vi "main.vi"(8 "error in (no error)":errorcluster, 11 "functional":refnum<user-event>) -> (0 "error out":errorcluster)   [LabVIEW 2015, in "functional.lvlib"]
uses:
  functional.lvlib
  _controls/event_functional.ctl
  _controls/event_functional_command.ctl
  private/_controls/event_common.ctl
  private/_controls/event_common_command.ctl
  private/_controls/event_interface.ctl
  private/_controls/event_interface_command.ctl
  _controls/hmi_references.ctl
  examples/example_01/functional/public/interface/interface.lvclass
  _controls/menu_selection.ctl
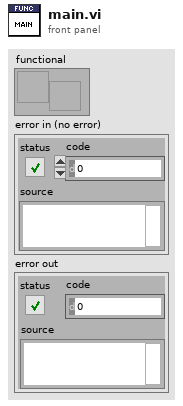
[diagram p1: front panel]
types:
  T1 = typedef "functional.lvlib/event_interface.ctl" = cluster{"command":T2, "data":variant}
  T2 = typedef "functional.lvlib/event_interface_command.ctl" = enum16{"<event_interface_cmd>", "<null>"}
  T3 = typedef "functional.lvlib/event_common.ctl" = cluster{"command":T4, "data":variant}
  T4 = typedef "functional.lvlib/event_common_command.ctl" = enum16{"<event_common_cmd>", "update_hmi_references", "die", "<null>"}
  T5 = cluster{"local":refnum<event-registration>, "external":refnum<event-registration>}
  T6 = typedef "functional.lvlib/hmi_references.ctl" = cluster{"vi_reference":refnum<vi>, "random_number":refnum<vi>, "do_it":refnum<vi>}
  T7 = cluster{"queue out":refnum<queue>, "example_01.lvlib:functional.lvlib:interface.lvclass":refnum<class "interface.lvclass">}
  T8 = typedef "functional.lvlib/event_functional.ctl" = cluster{"command":T9, "data":variant}
  T9 = typedef "functional.lvlib/event_functional_command.ctl" = enum16{"<command_functional>", "--high-level", "stop", "update_hmi_references", "load_interface", "--functional", "do_it", "<null>"}
  T10 = typedef "functional.lvlib/menu_selection.ctl" = enum16{"<menu>", "file_exit", "help_about", "<null>"}
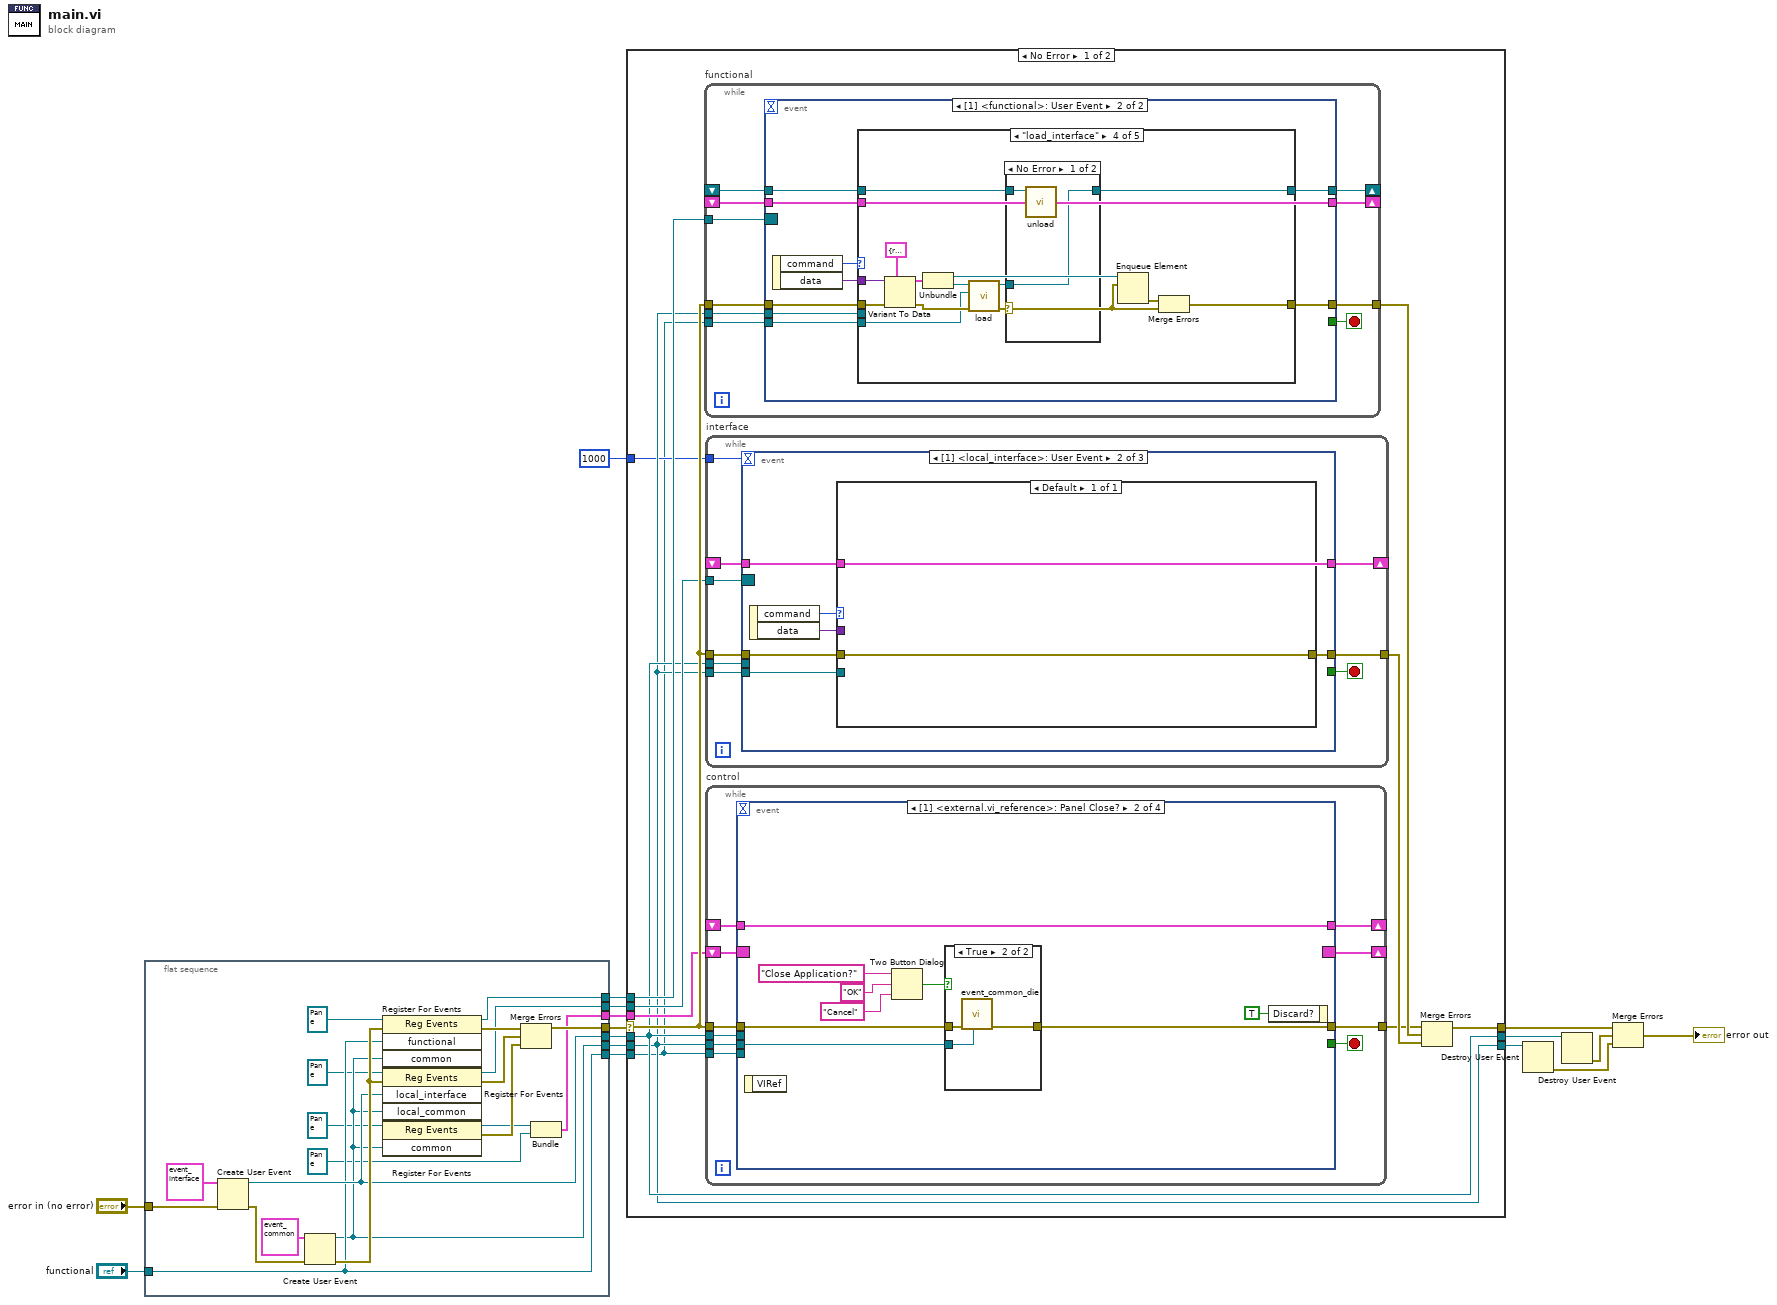
[diagram p0: block diagram]
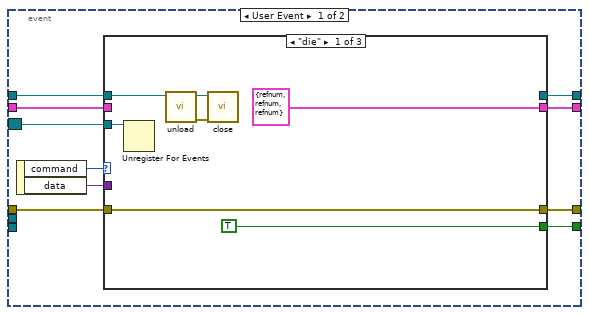
[diagram p2: hidden frame]
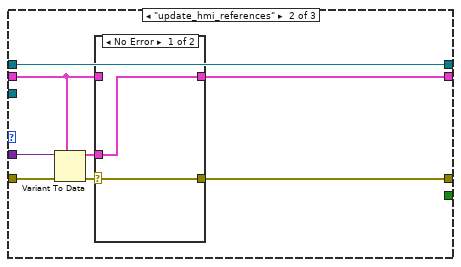
[diagram p3: hidden frame]
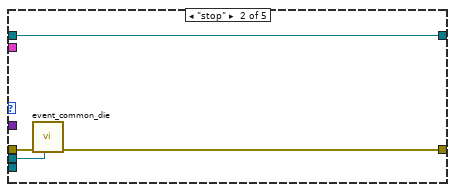
[diagram p7: hidden frame]
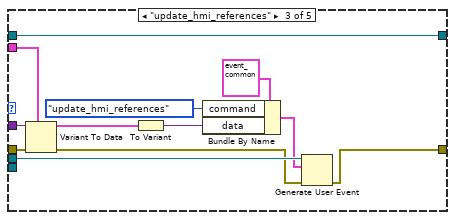
[diagram p8: hidden frame]
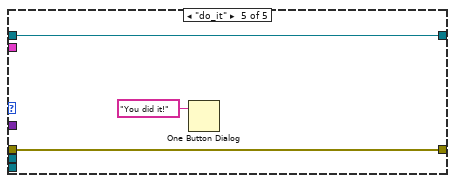
[diagram p10: hidden frame]
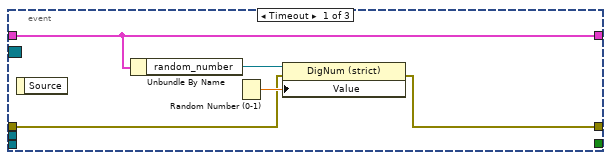
[diagram p11: hidden frame]
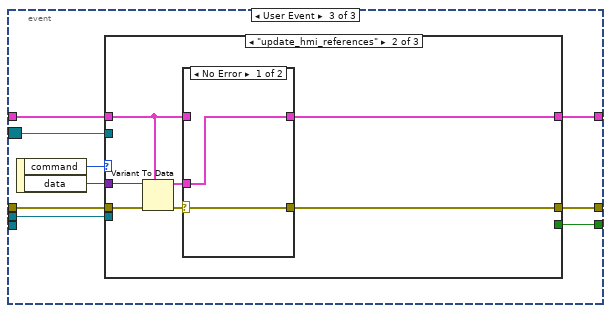
[diagram p12: hidden frame]
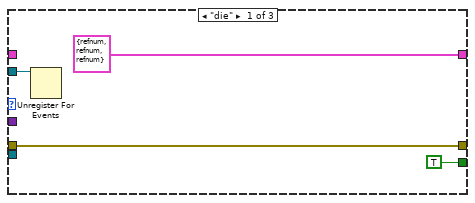
[diagram p13: hidden frame]
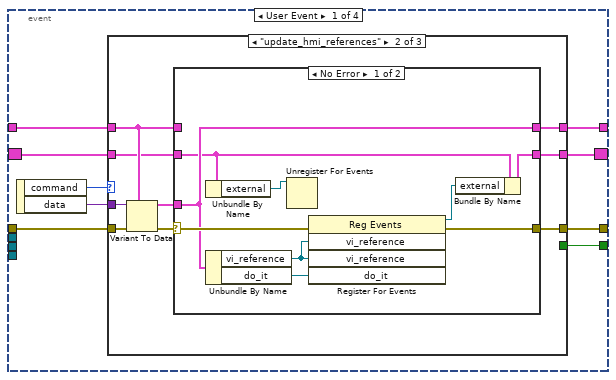
[diagram p16: hidden frame]
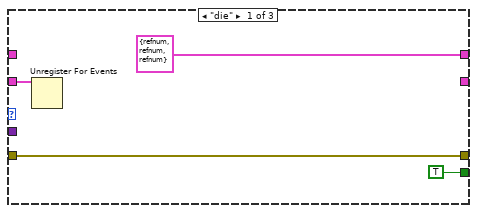
[diagram p17: hidden frame]
diagram:
  n1 = flat-sequence {
    tunnel: [w31] -> w16
    tunnel: [w21] -> w15
    tunnel: "error in (no error)" -> [w26]
    tunnel: [w30] -> w13
    tunnel: [w23] -> w11
    tunnel: [w27] -> w12
    tunnel: "functional" -> [w25]
    tunnel: [w25] -> w3
    tunnel: [w24] -> w2
    frame #0 {
      n2 = Create User Event(user event datatype=T1 {"command"=enum."<event_interface_cmd>", "data"=variant} ("interface"), error in=w26) -> (user event=w27:refnum<user-event>, error out=w32:errorcluster)
      n3 = Create User Event(user event datatype=T3 {"command"=enum."<event_common_cmd>", "data"=variant} ("common"), error in=w32) -> (user event=w23:refnum<user-event>, error out=w33:errorcluster)
      n4 = register-events(reference=refnum<event-registration> refnum ("local"), error in=w33, w25, w23) -> (reference out=w24:refnum<event-registration>, error out=w34:errorcluster)
      n5 = register-events(reference=refnum<event-registration> refnum ("local"), error in=w33, w27, w23) -> (reference out=w30:refnum<event-registration>, error out=w35:errorcluster)
      n6 = register-events(reference=refnum<event-registration> refnum ("local"), w23) -> (reference out=w22:refnum<event-registration>, error out=w36:errorcluster)  [unwired: 1 in]
      n7 = Merge Errors(w34, w35, w36) -> (w31:errorcluster)
      n8 = Bundle("local"=w22, "external"=refnum<event-registration> refnum) -> (w21:T5)  [unwired: 1 in]
    }
  }
  n9 = case shown="No Error" w16 {
    selector: w16 -> [w47 w279]
    tunnel: w15 -> [w45 w275]
    tunnel: [w43 w279] -> w8
    tunnel: w13 -> [w44 w276]
    tunnel: w12 -> [w42 w278]
    tunnel: w11 -> [w41 w277]
    tunnel: [w42 w278] -> w9
    tunnel: [w41 w277] -> w10
    tunnel: w3 -> [w37 _]
    tunnel: w2 -> [w48 w274]
    tunnel: 1000 -> [w38 _]
    frame No Error {
      n10 = while "functional" {
        tunnel: [w58] -> w40
        tunnel: w47 -> [w57]
        tunnel: w48 -> [w56]
        tunnel: w41 -> [w53]
        shift-right: [w52] -> _
        shift-left: _ -> [w55]
        tunnel: w37 -> [w51]
        shift-right: [w49] -> _
        shift-left: _ -> [w50]
        stop <- w54 stop-if-true
        n11 = event shown="[1] <functional>: User Event" {
          selector: w56 -> [w68 _]
          dyn-events: _ -> [_ _]
          timeout: _ -> [_ _]
          tunnel: [w65 w96] -> w58
          tunnel: w57 -> [w66 w97]
          tunnel: w55 -> [w62 w94]
          tunnel: [w64 _] -> w54
          tunnel: w53 -> [_ w95]
          tunnel: [w61 w94] -> w52
          tunnel: w51 -> [_ w93]
          tunnel: w50 -> [w60 w92]
          tunnel: [w59 w91] -> w49
          event User Event {
            n12 = event-data() -> ("command"=w67:T4, "data"=w63:variant)  [unwired: 1 in]
            n13 = case shown="\"die\"" w67 {
              tunnel: w66 -> [w74 w82 w90]
              tunnel: [w74 w80 w90] -> w65
              tunnel: [TRUE _ _] -> w64
              tunnel: w68 -> [w73 _ _]
              tunnel: w63 -> [_ w83 _]
              tunnel: w62 -> [_ w79 w89]
              tunnel: [T6 {"vi_reference"=refnum, "random_number"=refnum, "do_it"=refnum} ("hmi_references") w77 w89] -> w61
              tunnel: w60 -> [w71 w76 w88]
              tunnel: [_ w76 w88] -> w59
              frame "die" {
                n14 = Unregister For Events(event registration refnum=w73) -> ()  [unwired: 1 in, 1 out]
                n15 = call-dynamic "unload.vi"("interface in"=w71) -> ("error out"=w69:errorcluster, "interface out"=w70:refnum<class "interface.lvclass">)  [unwired: 9 in]
                n16 = call-dynamic "close.vi"("error in (no error)"=w69, "interface in"=w70) -> ()  [unwired: 8 in, 2 out]
              }
              frame "update_hmi_references" {
                n17 = Variant To Data(error in=w82, type=w79, Variant=w83) -> (data=w78:T6, error out=w81:errorcluster)
                n18 = case shown="No Error" w81 {
                  selector: w81 -> [w85 w87]
                  tunnel: [w85 w87] -> w80
                  tunnel: w79 -> [_ w86]
                  tunnel: w78 -> [w84 _]
                  tunnel: [w84 w86] -> w77
                  frame No Error {
                  }
                  frame Error {
                  }
                }
              }
              frame Default {
              }
            }
          }
          event User Event {
            n19 = event-data() -> ("command"=w98:T9, "data"=w99:variant)  [unwired: 1 in]
            n20 = case shown="\"load_interface\"" w98 {
              tunnel: w99 -> [_ _ w112 w130 _]
              tunnel: w97 -> [w101 w103 w117 w131 w137]
              tunnel: [w101 w102 w114 w122 w137] -> w96
              tunnel: w95 -> [_ w104 w116 _ _]
              tunnel: w94 -> [_ _ w113 _ _]
              tunnel: w93 -> [_ _ _ w127 _]
              tunnel: w92 -> [w100 w105 w106 w126 w135]
              tunnel: [w100 w105 w106 w118 w135] -> w91
              frame Default {
              }
              frame "stop" {
                n21 = call "event_common_die.vi"("local_common"=w104, "error in (no error)"=w103) -> ("error out"=w102:errorcluster)  [unwired: 9 in]
              }
              frame "update_hmi_references" {
                n22 = Variant To Data(error in=w117, type=w113, Variant=w112) -> (data=w109:T6, error out=w115:errorcluster)
                n23 = To Variant(anything=w109) -> (Variant=w107:variant)
                n24 = Bundle By Name(cluster=T3 {"command"=enum."<event_common_cmd>", "data"=variant} ("event data"), "command"=event_common_command."update_hmi_references", "data"=w107) -> (w110:T3)
                n25 = Generate User Event(user event=w116, event data cluster=w110, error in=w115) -> (error out=w114:errorcluster)  [unwired: 1 in, 1 out]
              }
              frame "load_interface" {
                n26 = Variant To Data(error in=w131, type=T7 {"queue out"=refnum, "example_01.lvlib:functional.lvlib:interface.lvclass"=refnum}, Variant=w130) -> (data=w129:T7, error out=w128:errorcluster)
                n27 = Unbundle(w129) -> ("queue out"=w123:refnum<queue>, "example_01.lvlib:functional.lvlib:interface.lvclass"=w124:refnum<class "interface.lvclass">)
                n28 = call-dynamic "load.vi"("error in (no error)"=w128, "functional"=w127, "interface in"=w124) -> ("error out"=w120:errorcluster, "interface out"=w119:refnum<class "interface.lvclass">)  [unwired: 7 in]
                n29 = case shown="No Error" w120 {
                  tunnel: w126 -> [w133 w134]
                  tunnel: w119 -> [w132 _]
                  tunnel: [w132 w134] -> w118
                  frame No Error {
                    n30 = call-dynamic "unload.vi"("interface in"=w133) -> ()  [unwired: 9 in, 2 out]
                  }
                  frame Error {
                  }
                }
                n31 = Enqueue Element(queue=w123, element=w120) -> (error out=w121:errorcluster)  [unwired: 2 in, 2 out]
                n32 = Merge Errors(w121, w120) -> (w122:errorcluster)
              }
              frame "do_it" {
                n33 = One Button Dialog(message="You did it!") -> ()  [unwired: 1 in, 1 out]
              }
            }
          }
        }
      }
      n34 = while "interface" {
        tunnel: w47 -> [w146]
        tunnel: [w144] -> w46
        tunnel: w44 -> [w143]
        tunnel: w42 -> [w138]
        tunnel: w41 -> [w142]
        shift-right: [w140] -> _
        shift-left: _ -> [w141]
        tunnel: w38 -> [w139]
        stop <- w145 stop-if-true
        n35 = event shown="[1] <local_interface>: User Event" {
          selector: w143 -> [_ _ w163]
          dyn-events: _ -> [_ _ _]
          timeout: w139 -> [_ _ _]
          tunnel: w146 -> [w148 w155 w166]
          tunnel: [w147 w154 w165] -> w144
          tunnel: [_ _ w164] -> w145
          tunnel: w142 -> [_ w153 _]
          tunnel: w141 -> [w149 w152 w161]
          tunnel: [w149 w152 w160] -> w140
          tunnel: w138 -> [_ _ w159]
          event Timeout {
            n36 = event-data() -> ()  [unwired: 1 in, 1 out]
            n37 = Unbundle By Name(w149) -> ("random_number"=w151:refnum<vi>)
            n38 = Random Number (0-1)() -> (number: 0 to 1=w150:dbl)
            n39 = property class="DigNum (strict)"(reference=w151, error in=w148, "Value"=w150) -> (error out=w147:errorcluster)  [unwired: 1 out]
          }
          event User Event {
            n40 = event-data() -> ("command"=w157:T2, "data"=w156:variant)  [unwired: 1 in]
            n41 = case shown="Default" w157 {
              tunnel: w155 -> [w158]
              tunnel: [w158] -> w154
              tunnel: w156 -> [_]
              tunnel: w153 -> [_]
              tunnel: w152 -> [_]
              frame Default {
              }
            }
          }
          event User Event {
            n42 = event-data() -> ("command"=w167:T4, "data"=w162:variant)  [unwired: 1 in]
            n43 = case shown="\"update_hmi_references\"" w167 {
              tunnel: w166 -> [w170 w175 w184]
              tunnel: [w170 w172 w184] -> w165
              tunnel: [TRUE _ _] -> w164
              tunnel: w163 -> [w169 _ _]
              tunnel: w162 -> [_ w174 _]
              tunnel: w161 -> [_ w176 w183]
              tunnel: [T6 {"vi_reference"=refnum, "random_number"=refnum, "do_it"=refnum} ("hmi_references") w173 w183] -> w160
              tunnel: w159 -> [_ _ _]
              frame "die" {
                n44 = Unregister For Events(event registration refnum=w169) -> ()  [unwired: 1 in, 1 out]
              }
              frame "update_hmi_references" {
                n45 = Variant To Data(error in=w175, type=w176, Variant=w174) -> (data=w177:T6, error out=w178:errorcluster)
                n46 = case shown="No Error" w178 {
                  selector: w178 -> [w179 w182]
                  tunnel: [w179 w182] -> w172
                  tunnel: w176 -> [_ w181]
                  tunnel: w177 -> [w180 _]
                  tunnel: [w180 w181] -> w173
                  frame No Error {
                  }
                  frame Error {
                  }
                }
              }
              frame Default {
              }
            }
          }
        }
      }
      n47 = while "control" {
        tunnel: w47 -> [w194]
        tunnel: [w192] -> w39
        tunnel: w42 -> [w189]
        tunnel: w41 -> [w188]
        shift-right: [w187] -> _
        shift-left: _ -> [w190]
        shift-right: [w186] -> _
        shift-left: w45 -> [w191]
        tunnel: w37 -> [w185]
        stop <- w193 stop-if-true
        n48 = event shown="[1] <external.vi_reference>: Panel Close?" {
          selector: w191 -> [w198 _ _ _]
          dyn-events: [w195 _ _ _] -> w186
          timeout: _ -> [_ _ _ _]
          tunnel: w194 -> [w202 w234 w247 w254]
          tunnel: [w201 w239 w246 w252] -> w192
          tunnel: [w200 _ _ _] -> w193
          tunnel: w190 -> [w197 w233 w249 w251]
          tunnel: w189 -> [_ _ _ _]
          tunnel: w188 -> [_ w232 _ w250]
          tunnel: [w196 w233 w249 w251] -> w187
          tunnel: w185 -> [_ _ w248 _]
          event User Event {
            n49 = event-data() -> ("command"=w203:T4, "data"=w199:variant)  [unwired: 1 in]
            n50 = case shown="\"update_hmi_references\"" w203 {
              tunnel: w202 -> [w205 w212 w231]
              tunnel: [w205 w210 w231] -> w201
              tunnel: [TRUE _ _] -> w200
              tunnel: w199 -> [_ w214 _]
              tunnel: w198 -> [w206 w209 w230]
              tunnel: w197 -> [_ w213 w229]
              tunnel: [T6 {"vi_reference"=refnum, "random_number"=refnum, "do_it"=refnum} ("hmi_references") w211 w229] -> w196
              tunnel: [_ w208 w230] -> w195
              frame "die" {
                n51 = Unregister For Events(event registration refnum=w206) -> ()  [unwired: 1 in, 1 out]
              }
              frame "update_hmi_references" {
                n52 = Variant To Data(error in=w212, type=w213, Variant=w214) -> (data=w216:T6, error out=w215:errorcluster)
                n53 = case shown="No Error" w215 {
                  selector: w215 -> [w223 w228]
                  tunnel: [w222 w228] -> w210
                  tunnel: w213 -> [_ w227]
                  tunnel: w216 -> [w220 _]
                  tunnel: [w220 w227] -> w211
                  tunnel: w209 -> [w218 w226]
                  tunnel: [w225 w226] -> w208
                  frame No Error {
                    n54 = Unbundle By Name(w218) -> ("external"=w217:refnum<event-registration>)
                    n55 = Unbundle By Name(w220) -> ("vi_reference"=w219:refnum<vi>, "do_it"=w224:refnum<vi>)
                    n56 = Unregister For Events(event registration refnum=w217) -> ()  [unwired: 1 in, 1 out]
                    n57 = register-events(error in=w223, w219, w219, w224) -> (reference out=w221:refnum<event-registration>, error out=w222:errorcluster)  [unwired: 1 in]
                    n58 = Bundle By Name(cluster=w218, "external"=w221) -> (w225:T5)
                  }
                  frame Error {
                  }
                }
              }
              frame Default {
              }
            }
          }
          event Panel Close? {
            n59 = event-data() -> ()  [unwired: 1 in, 1 out]
            n60 = Two Button Dialog(message="Close Application?" ("dialog_text"), 1:"Cancel" ("boolean_text_1"), 2:"OK" ("boolean_text_1")) -> (T button?=w235:bool)
            n61 = case shown="True" w235 {
              tunnel: w234 -> [w241 w243]
              tunnel: [w241 w242] -> w239
              tunnel: w232 -> [_ w244]
              frame False {
              }
              frame True {
                n62 = call "event_common_die.vi"("local_common"=w244, "error in (no error)"=w243) -> ("error out"=w242:errorcluster)  [unwired: 9 in]
              }
            }
            n63 = event-data("Discard?"=TRUE) -> ()  [unwired: 1 in, 1 out]
          }
          event Value Change {
            n64 = event-data() -> ()  [unwired: 1 in, 1 out]
            n65 = Generate User Event(user event=w248, event data cluster=T8 {"command"=enum."do_it", "data"=variant} ("event data"), error in=w247) -> (error out=w246:errorcluster)  [unwired: 1 in, 1 out]
          }
          event Menu Selection (User) {
            n66 = event-data() -> ("MenuRef"=w255:refnum<k9>, "ItemTag"=w253:string)  [unwired: 1 in]
            n67 = Scan From String(input string=w253, default 1=menu_selection."<menu>" ("menu_selection")) -> (output 1=w256:T10)  [unwired: 3 in, 3 out]
            n68 = case shown="\"file_exit\"" w256 {
              tunnel: w255 -> [_ _]
              tunnel: w254 -> [w258 w263]
              tunnel: w253 -> [w262 _]
              tunnel: [w258 w269] -> w252
              tunnel: w250 -> [_ w268]
              frame Default {
                n69 = Format Into String(format string="Invalid Menu Option Selected: %s.", w262) -> (resulting string=w260:string)  [unwired: 2 in, 1 out]
                n70 = One Button Dialog(message=w260, button name ("OK")="OK" ("boolean_text_1")) -> ()  [unwired: 1 out]
              }
              frame "file_exit" {
                n71 = Two Button Dialog(message="Close Application?" ("dialog_text"), 1:"Cancel" ("boolean_text_1"), 2:"OK" ("boolean_text_1")) -> (T button?=w264:bool)
                n72 = case shown="False" w264 {
                  tunnel: w263 -> [w270 w273]
                  tunnel: [w270 w272] -> w269
                  tunnel: w268 -> [_ w271]
                  frame False {
                  }
                  frame True {
                    n73 = call "event_common_die.vi"("local_common"=w271, "error in (no error)"=w273) -> ("error out"=w272:errorcluster)  [unwired: 9 in]
                  }
                }
              }
            }
          }
        }
      }
      n74 = Merge Errors(w39, w40, w46) -> (w43:errorcluster)
    }
    frame Error {
      n75 = Unregister For Events(event registration refnum=w276) -> ()  [unwired: 1 in, 1 out]
      n76 = Unregister For Events(event registration refnum=w275) -> ()  [unwired: 1 in, 1 out]
      n77 = Unregister For Events(event registration refnum=w274) -> ()  [unwired: 1 in, 1 out]
    }
  }
  n78 = Destroy User Event(user event=w10) -> (error out=w6:errorcluster)  [unwired: 1 in]
  n79 = Destroy User Event(user event=w9) -> (error out=w7:errorcluster)  [unwired: 1 in]
  n80 = Merge Errors(w8, w7, w6) -> (→"error out":errorcluster)
